vi "Parse Accept Header.vi"(11 "Accept Value":string) -> (3 "Media Types":T1[](array[typedef]))   [LabVIEW 2020, in "CSM WebService.lvlib"]
doc: "Parses the value of the HTTP Accept header sent by a client and produces an ordered array of the media types that the client accepts.\n\nThe Accept header is a comma-separated list of type/subtype values. A * for either the type or subtype represents a wildcard that matches anything. After each subtype, there is optionally a semicolon-separated list of parameters. Each parameter may or may not have a value in the form parameter=value or parameter=\"value\". In the case where the value is quoted, there may be escaped characters, including another quote, using a backslash. Once parsed, the correct order is determined in Sort Media Types.vi.\n\nExample: text/xml; q=0.5, image/jpeg; q=0.8, image/png; q=0.8; version=5, text/*, image/*, */*; q=1\n\nproduces the following order: image/png, image/jpeg, text/xml, text/*, image/*, */*"
uses:
  CSM WebService.lvlib
  Accept State.ctl
  Media Parameter.ctl
  Media Type.ctl
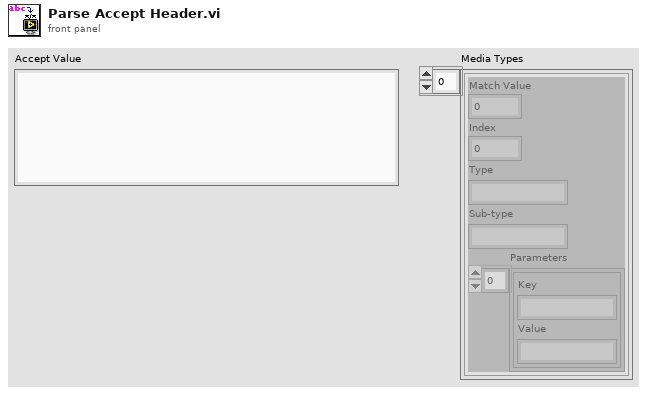
[diagram p1: front panel]
types:
  T1 = typedef "CSM WebService.lvlib/Media Type.ctl" = cluster{"Match Value":dbl, "Index":i32, "Type":string, "Sub-type":string, "Parameters":T2[]}
  T2 = typedef "CSM WebService.lvlib/Media Parameter.ctl" = cluster{"Key":string, "Value":string}
  T3 = typedef "CSM WebService.lvlib/Accept State.ctl" = enum16{"Type", "Sub-type", "Parameter", "Value", "Quoted Value", "Escaped Character"}
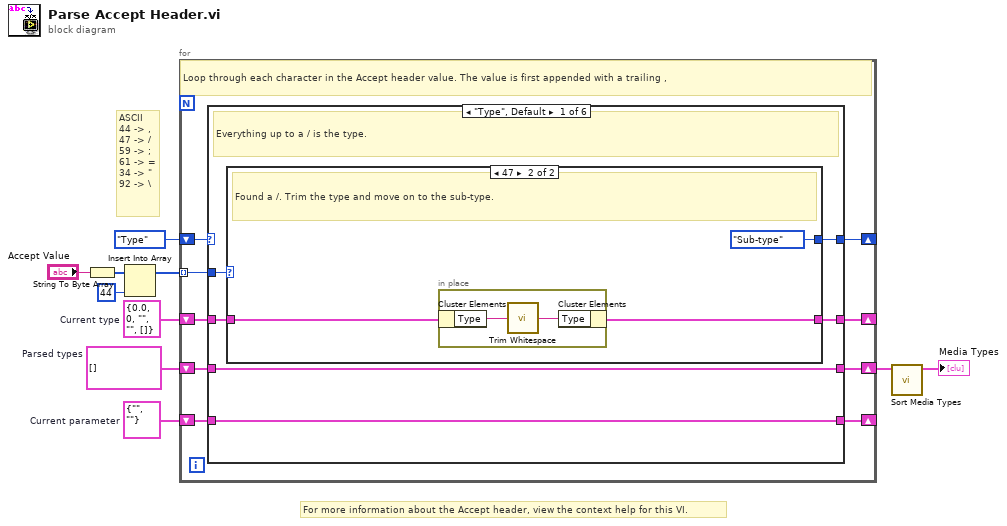
[diagram p0: block diagram]
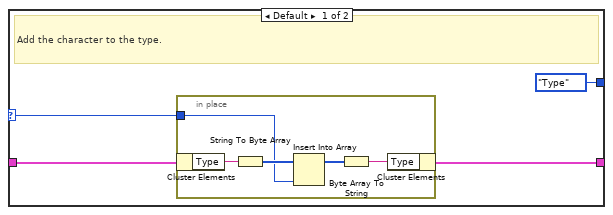
[diagram p2: hidden frame]
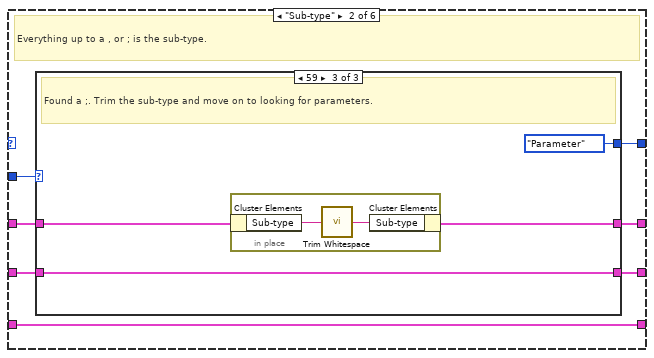
[diagram p3: hidden frame]
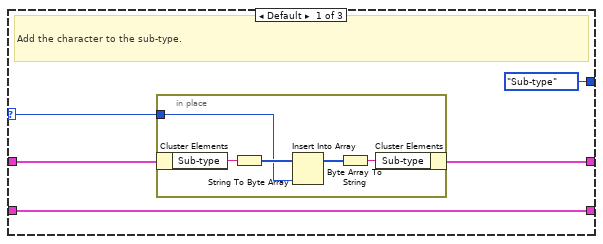
[diagram p4: hidden frame]
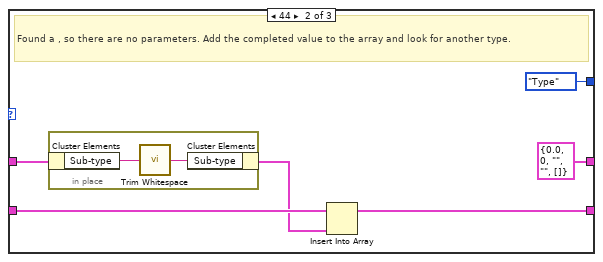
[diagram p5: hidden frame]
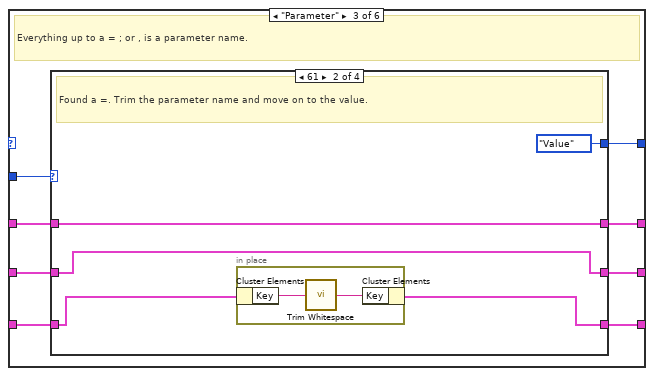
[diagram p6: hidden frame]
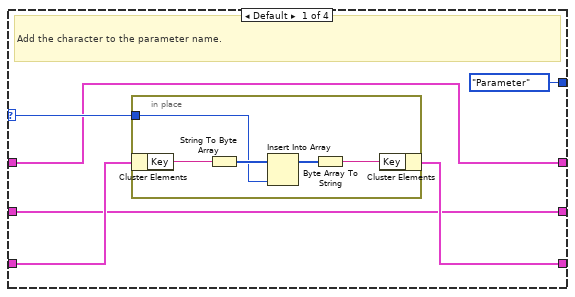
[diagram p7: hidden frame]
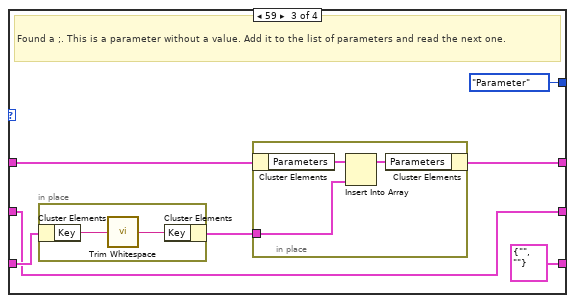
[diagram p8: hidden frame]
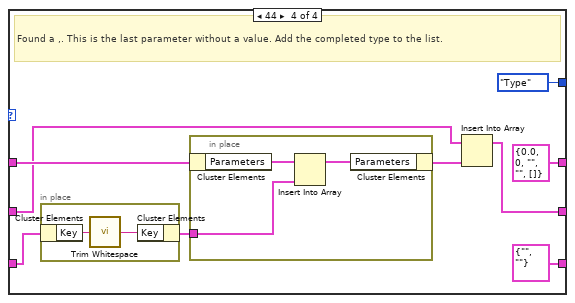
[diagram p9: hidden frame]
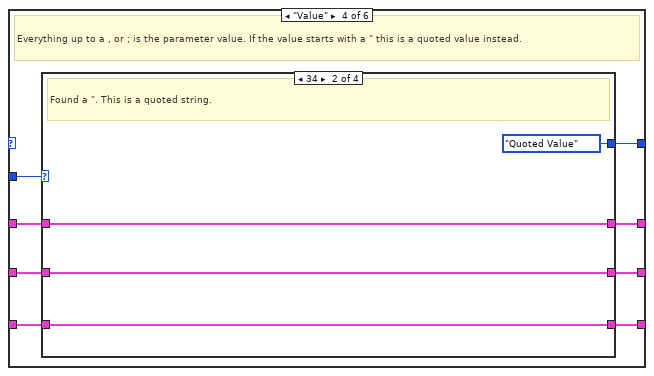
[diagram p10: hidden frame]
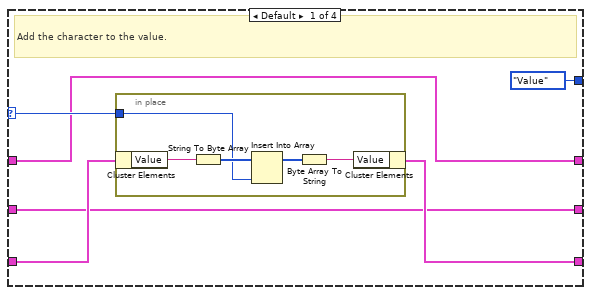
[diagram p11: hidden frame]
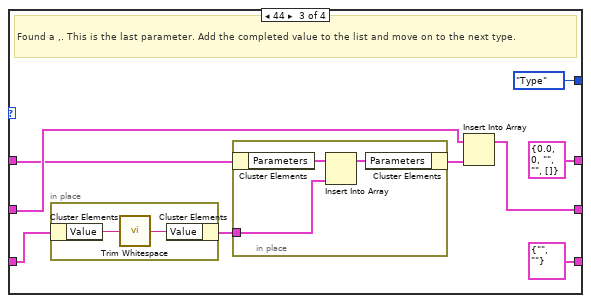
[diagram p12: hidden frame]
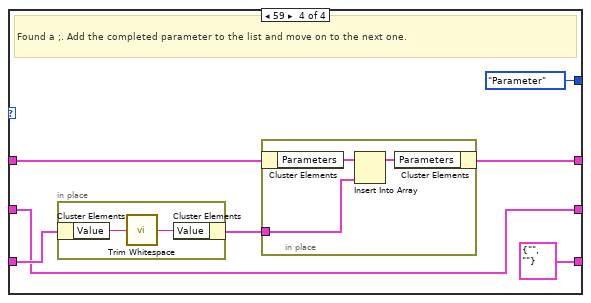
[diagram p13: hidden frame]
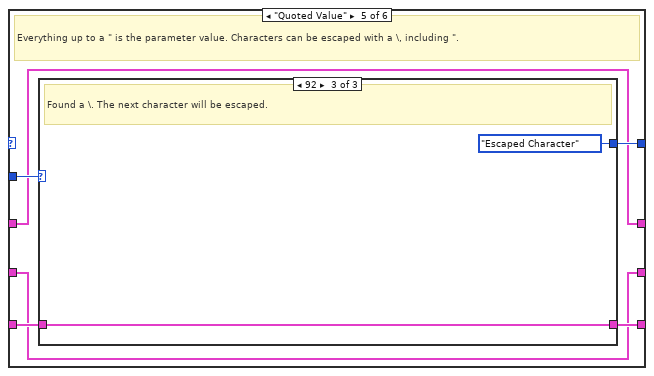
[diagram p14: hidden frame]
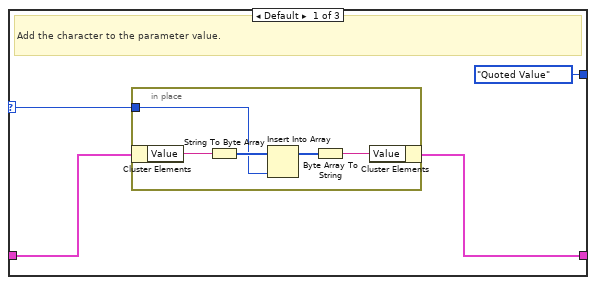
[diagram p15: hidden frame]
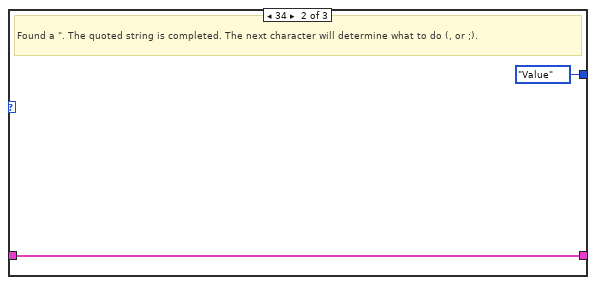
[diagram p16: hidden frame]
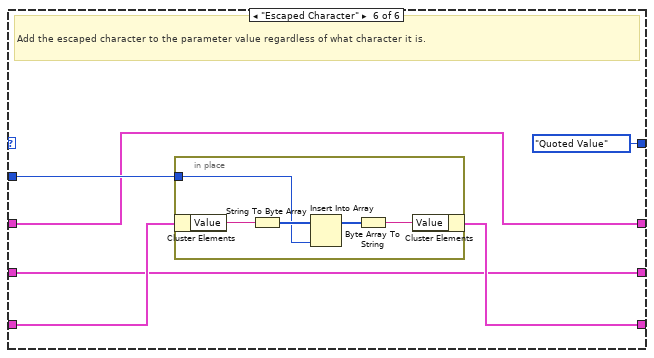
[diagram p17: hidden frame]
diagram:
  w9 = T2 {"Key"="", "Value"=""}  # Current parameter
  w8 = T1 {"Match Value"=0.0, "Index"=0, "Type"="", "Sub-type"="", "Parameters"=[]}  # Current type
  w7 = T1[] []  # Parsed types
  # "ASCII\n44 -> ,\n47 -> /\n59 -> ;\n61 -> =\n34 -> \"\n92 -> \\"
  # "For more information about the Accept header, view the context help for this VI."
  n1 = String To Byte Array(string="Accept Value") -> (unsigned byte array=w5:u8[])
  n2 = Insert Into Array(array=w5, new element=u8 44 ("new element/subarray")) -> (w2:u8[])  [unwired: 1 in]
  n3 = for {
    tunnel: w2 -> [w18] mode=indexing
    shift-right: [w17] -> _
    shift-left: Accept_State."Type" -> [w19]
    shift-right: [w11] -> w10
    shift-left: w7 -> [w13]
    shift-right: [w15] -> _
    shift-left: w8 -> [w16]
    shift-right: [w12] -> _
    shift-left: w9 -> [w14]
    # "Loop through each character in the Accept header value. The value is first appended with a trailing ,"
    n4 = case shown="\"Type\", Default" w19 {
      tunnel: w18 -> [w25 w46 w78 w130 w177 w196]
      tunnel: [w24 w45 w77 w129 w175 Accept_State."Quoted Value"] -> w17
      tunnel: w16 -> [w23 w44 w74 w128 w172 w192]
      tunnel: [w22 w43 w73 w125 w172 w192] -> w15
      tunnel: w14 -> [w21 w42 w76 w126 w176 w195]
      tunnel: w13 -> [w20 w41 w72 w127 w173 w193]
      tunnel: [w21 w42 w75 w123 w174 w194] -> w12
      tunnel: [w20 w40 w71 w124 w173 w193] -> w11
      frame "Type", Default {
        # "Everything up to a / is the type."
        n5 = case shown="47" w25 {
          selector: w25 -> [w27 _]
          tunnel: [Accept_State."Type" Accept_State."Sub-type"] -> w24
          tunnel: w23 -> [w28 w36]
          tunnel: [w26 w35] -> w22
          frame Default {
            # "Add the character to the type."
            n6 = in-place {
              in-place-border: w27 -> [w32]
              n7 = in-place-cluster #1(w28) -> ("Type"=w34:string)
              n8 = String To Byte Array(string=w34) -> (unsigned byte array=w33:u8[])
              n9 = Insert Into Array(array=w33, new element=w32) -> (w31:u8[])  [unwired: 1 in]
              n10 = Byte Array To String(unsigned byte array=w31) -> (string=w30:string)
              n11 = in-place-cluster #1("Type"=w30) -> (w26:T1)
            }
          }
          frame 47 {
            # "Found a /. Trim the type and move on to the sub-type."
            n12 = in-place {
              n13 = in-place-cluster #2(w36) -> ("Type"=w39:string)
              n14 = call <vilib>:"Trim Whitespace.vi"("string"=w39) -> ("trimmed string"=w38:string)  [unwired: 1 in]
              n15 = in-place-cluster #2("Type"=w38) -> (w35:T1)
            }
          }
        }
      }
      frame "Sub-type" {
        # "Everything up to a , or ; is the sub-type."
        n16 = case shown="59" w46 {
          selector: w46 -> [w50 _ _]
          tunnel: [Accept_State."Sub-type" Accept_State."Type" Accept_State."Parameter"] -> w45
          tunnel: w44 -> [w49 w61 w67]
          tunnel: [w48 T1 {"Match Value"=0.0, "Index"=0, "Type"="", "Sub-type"="", "Parameters"=[]} w66] -> w43
          tunnel: w41 -> [w47 w60 w65]
          tunnel: [w47 w59 w65] -> w40
          frame Default {
            # "Add the character to the sub-type."
            n17 = in-place {
              in-place-border: w50 -> [w54]
              n18 = in-place-cluster #3(w49) -> ("Sub-type"=w56:string)
              n19 = String To Byte Array(string=w56) -> (unsigned byte array=w55:u8[])
              n20 = Insert Into Array(array=w55, new element=w54) -> (w53:u8[])  [unwired: 1 in]
              n21 = Byte Array To String(unsigned byte array=w53) -> (string=w52:string)
              n22 = in-place-cluster #3("Sub-type"=w52) -> (w48:T1)
            }
          }
          frame 44 {
            # "Found a , so there are no parameters. Add the completed value to the array and look for another type."
            n23 = in-place {
              n24 = in-place-cluster #4(w61) -> ("Sub-type"=w64:string)
              n25 = call <vilib>:"Trim Whitespace.vi"("string"=w64) -> ("trimmed string"=w63:string)  [unwired: 1 in]
              n26 = in-place-cluster #4("Sub-type"=w63) -> (w58:T1)
            }
            n27 = Insert Into Array(array=w60, new element=w58) -> (w59:T1[])  [unwired: 1 in]
          }
          frame 59 {
            # "Found a ;. Trim the sub-type and move on to looking for parameters."
            n28 = in-place {
              n29 = in-place-cluster #5(w67) -> ("Sub-type"=w70:string)
              n30 = call <vilib>:"Trim Whitespace.vi"("string"=w70) -> ("trimmed string"=w69:string)  [unwired: 1 in]
              n31 = in-place-cluster #5("Sub-type"=w69) -> (w66:T1)
            }
          }
        }
      }
      frame "Parameter" {
        # "Everything up to a = ; or , is a parameter name."
        n32 = case shown="61" w78 {
          selector: w78 -> [w83 _ _ _]
          tunnel: [Accept_State."Parameter" Accept_State."Value" Accept_State."Parameter" Accept_State."Type"] -> w77
          tunnel: w76 -> [w82 w93 w102 w115]
          tunnel: [w81 w92 T2 {"Key"="", "Value"=""} ("Parameter") T2 {"Key"="", "Value"=""} ("Parameter")] -> w75
          tunnel: w74 -> [w79 w91 w101 w114]
          tunnel: [w79 w91 w98 T1 {"Match Value"=0.0, "Index"=0, "Type"="", "Sub-type"="", "Parameters"=[]}] -> w73
          tunnel: w72 -> [w80 w90 w97 w111]
          tunnel: [w80 w90 w97 w110] -> w71
          frame Default {
            # "Add the character to the parameter name."
            n33 = in-place {
              in-place-border: w83 -> [w87]
              n34 = in-place-cluster #6(w82) -> ("Key"=w89:string)
              n35 = String To Byte Array(string=w89) -> (unsigned byte array=w88:u8[])
              n36 = Insert Into Array(array=w88, new element=w87) -> (w86:u8[])  [unwired: 1 in]
              n37 = Byte Array To String(unsigned byte array=w86) -> (string=w85:string)
              n38 = in-place-cluster #6("Key"=w85) -> (w81:T2)
            }
          }
          frame 61 {
            # "Found a =. Trim the parameter name and move on to the value."
            n39 = in-place {
              n40 = in-place-cluster #7(w93) -> ("Key"=w96:string)
              n41 = call <vilib>:"Trim Whitespace.vi"("string"=w96) -> ("trimmed string"=w95:string)  [unwired: 1 in]
              n42 = in-place-cluster #7("Key"=w95) -> (w92:T2)
            }
          }
          frame 59 {
            # "Found a ;. This is a parameter without a value. Add it to the list of parameters and read the next one."
            n43 = in-place {
              n44 = in-place-cluster #8(w102) -> ("Key"=w108:string)
              n45 = call <vilib>:"Trim Whitespace.vi"("string"=w108) -> ("trimmed string"=w107:string)  [unwired: 1 in]
              n46 = in-place-cluster #8("Key"=w107) -> (w100:T2)
            }
            n47 = in-place {
              in-place-border: w100 -> [w105]
              n48 = in-place-cluster #9(w101) -> ("Parameters"=w106:T2[])
              n49 = Insert Into Array(array=w106, new element=w105) -> (w104:T2[])  [unwired: 1 in]
              n50 = in-place-cluster #9("Parameters"=w104) -> (w98:T1)
            }
          }
          frame 44 {
            # "Found a ,. This is the last parameter without a value. Add the completed type to the list."
            n51 = in-place {
              n52 = in-place-cluster #10(w115) -> ("Key"=w122:string)
              n53 = call <vilib>:"Trim Whitespace.vi"("string"=w122) -> ("trimmed string"=w121:string)  [unwired: 1 in]
              n54 = in-place-cluster #10("Key"=w121) -> (w116:T2)
            }
            n55 = in-place {
              in-place-border: w116 -> [w118]
              n56 = in-place-cluster #11(w114) -> ("Parameters"=w120:T2[])
              n57 = Insert Into Array(array=w120, new element=w118) -> (w119:T2[])  [unwired: 1 in]
              n58 = in-place-cluster #11("Parameters"=w119) -> (w112:T1)
            }
            n59 = Insert Into Array(array=w111, new element=w112) -> (w110:T1[])  [unwired: 1 in]
          }
        }
      }
      frame "Value" {
        # "Everything up to a , or ; is the parameter value. If the value starts with a \" this is a quoted value instead."
        n60 = case shown="34" w130 {
          selector: w130 -> [w135 _ _ _]
          tunnel: [Accept_State."Value" Accept_State."Quoted Value" Accept_State."Type" Accept_State."Parameter"] -> w129
          tunnel: w128 -> [w131 w144 w150 w164]
          tunnel: w127 -> [w132 w143 w151 w160]
          tunnel: w126 -> [w134 w142 w149 w161]
          tunnel: [w131 w144 T1 {"Match Value"=0.0, "Index"=0, "Type"="", "Sub-type"="", "Parameters"=[]} w163] -> w125
          tunnel: [w132 w143 w148 w160] -> w124
          tunnel: [w133 w142 T2 {"Key"="", "Value"=""} ("Parameter") T2 {"Key"="", "Value"=""} ("Parameter")] -> w123
          frame Default {
            # "Add the character to the value."
            n61 = in-place {
              in-place-border: w135 -> [w139]
              n62 = in-place-cluster #12(w134) -> ("Value"=w141:string)
              n63 = String To Byte Array(string=w141) -> (unsigned byte array=w140:u8[])
              n64 = Insert Into Array(array=w140, new element=w139) -> (w138:u8[])  [unwired: 1 in]
              n65 = Byte Array To String(unsigned byte array=w138) -> (string=w137:string)
              n66 = in-place-cluster #12("Value"=w137) -> (w133:T2)
            }
          }
          frame 34 {
            # "Found a \". This is a quoted string."
          }
          frame 44 {
            # "Found a ,. This is the last parameter. Add the completed value to the list and move on to the next type."
            n67 = in-place {
              n68 = in-place-cluster #13(w149) -> ("Value"=w159:string)
              n69 = call <vilib>:"Trim Whitespace.vi"("string"=w159) -> ("trimmed string"=w158:string)  [unwired: 1 in]
              n70 = in-place-cluster #13("Value"=w158) -> (w153:T2)
            }
            n71 = in-place {
              in-place-border: w153 -> [w156]
              n72 = in-place-cluster #14(w150) -> ("Parameters"=w157:T2[])
              n73 = Insert Into Array(array=w157, new element=w156) -> (w155:T2[])  [unwired: 1 in]
              n74 = in-place-cluster #14("Parameters"=w155) -> (w152:T1)
            }
            n75 = Insert Into Array(array=w151, new element=w152) -> (w148:T1[])  [unwired: 1 in]
          }
          frame 59 {
            # "Found a ;. Add the completed parameter to the list and move on to the next one."
            n76 = in-place {
              n77 = in-place-cluster #15(w161) -> ("Value"=w171:string)
              n78 = call <vilib>:"Trim Whitespace.vi"("string"=w171) -> ("trimmed string"=w170:string)  [unwired: 1 in]
              n79 = in-place-cluster #15("Value"=w170) -> (w165:T2)
            }
            n80 = in-place {
              in-place-border: w165 -> [w168]
              n81 = in-place-cluster #16(w164) -> ("Parameters"=w169:T2[])
              n82 = Insert Into Array(array=w169, new element=w168) -> (w167:T2[])  [unwired: 1 in]
              n83 = in-place-cluster #16("Parameters"=w167) -> (w163:T1)
            }
          }
        }
      }
      frame "Quoted Value" {
        # "Everything up to a \" is the parameter value. Characters can be escaped with a \\, including \"."
        n84 = case shown="92" w177 {
          selector: w177 -> [w180 _ _]
          tunnel: w176 -> [w179 w187 w189]
          tunnel: [Accept_State."Quoted Value" Accept_State."Value" Accept_State."Escaped Character"] -> w175
          tunnel: [w178 w187 w189] -> w174
          frame Default {
            # "Add the character to the parameter value."
            n85 = in-place {
              in-place-border: w180 -> [w184]
              n86 = in-place-cluster #17(w179) -> ("Value"=w186:string)
              n87 = String To Byte Array(string=w186) -> (unsigned byte array=w185:u8[])
              n88 = Insert Into Array(array=w185, new element=w184) -> (w183:u8[])  [unwired: 1 in]
              n89 = Byte Array To String(unsigned byte array=w183) -> (string=w182:string)
              n90 = in-place-cluster #17("Value"=w182) -> (w178:T2)
            }
          }
          frame 34 {
            # "Found a \". The quoted string is completed. The next character will determine what to do (, or ;)."
          }
          frame 92 {
            # "Found a \\. The next character will be escaped."
          }
        }
      }
      frame "Escaped Character" {
        # "Add the escaped character to the parameter value regardless of what character it is."
        n91 = in-place {
          in-place-border: w196 -> [w199]
          n92 = in-place-cluster #18(w195) -> ("Value"=w201:string)
          n93 = String To Byte Array(string=w201) -> (unsigned byte array=w200:u8[])
          n94 = Insert Into Array(array=w200, new element=w199) -> (w198:u8[])  [unwired: 1 in]
          n95 = Byte Array To String(unsigned byte array=w198) -> (string=w197:string)
          n96 = in-place-cluster #18("Value"=w197) -> (w194:T2)
        }
      }
    }
  }
  n97 = call "Sort Media Types.vi"("Parsed Types"=w10) -> ("Sorted types"=→"Media Types":T1[])  [unwired: 10 in]
